vi "Main.vi"() -> ()   [LabVIEW 2023]
uses:
  CONTROLS/Control 1.ctl
panel:
  out "Enum":T1
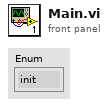
[diagram p1: front panel]
types:
  T1 = typedef "Control 1.ctl" = enum16{"init", "read", "write", "Kundeneingabe", "Betonauswahl", "Bezahlprozess", "Zutaten hinzufügen", "Zutaten mit Gewichtsmessung", "Stopp", "Gewicht", "Rechnung"}
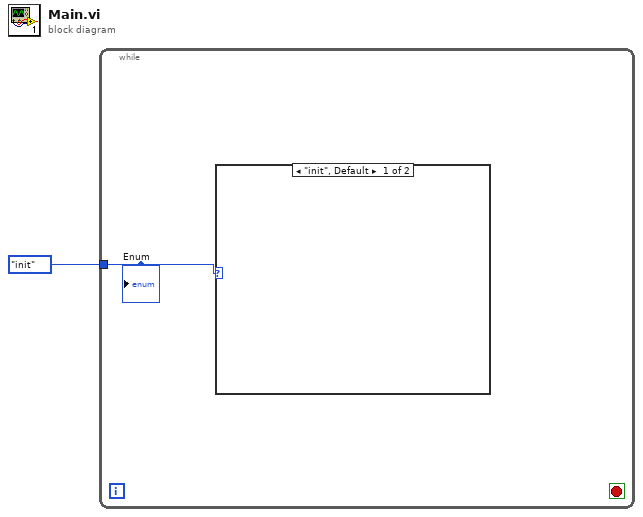
[diagram p0: block diagram]
diagram:
  n1 = while {
    tunnel: Control_1."init" -> [w2]
    stop <- _ stop-if-true
    n2 = case shown="\"init\", Default" w2 {
      frame "init", Default {
      }
      frame "read" {
      }
    }
    "Enum" <- w2
  }
